vi "Write Cell font.vi"(8 "error in (no error)":errorcluster, 10 "Font":T1, 11 "DatagridElement in":refnum<class "DatagridElement.lvclass">) -> (0 "error out":errorcluster, 3 "DatagridElement out":refnum<class "DatagridElement.lvclass">)   [LabVIEW 2023, in "D Datagrid Library.lvlib" / "DatagridElement.lvclass"]
uses:
  DatagridElement.lvclass
  <vilib>/Utility/miscctls.llb/LVFontTypeDef.ctl
  DatagridElement.lvclass/DatagridElement.ctl
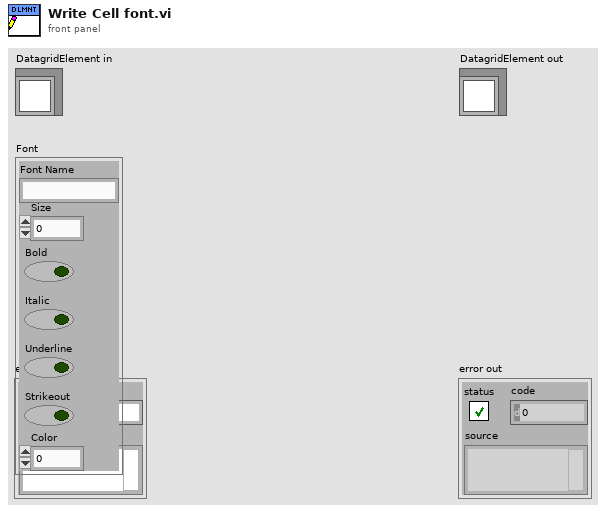
[diagram p1: front panel]
types:
  T1 = typedef "LVFontTypeDef.ctl" = cluster{"Font Name":string, "Size":u16, "Bold":bool, "Italic":bool, "Underline":bool, "Strikeout":bool, "Color":u32}
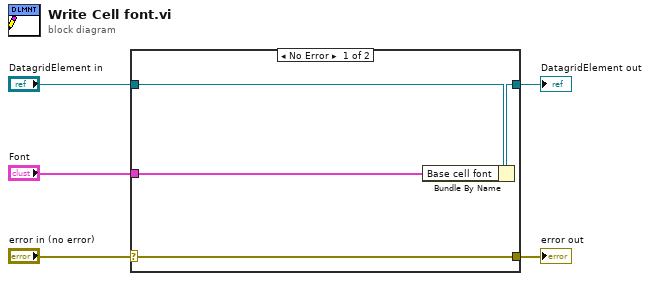
[diagram p0: block diagram]
diagram:
  n1 = case shown="No Error" "error in (no error)" {
    selector: "error in (no error)" -> [w9 w10]
    tunnel: [w9 w10] -> w4
    tunnel: [w7 w11] -> w2
    tunnel: "DatagridElement in" -> [w8 w11]
    tunnel: "Font" -> [w6 _]
    frame No Error {
      n2 = Bundle By Name(cluster=w8, "Base cell font"=w6) -> (w7:refnum<class "DatagridElement.lvclass">)
    }
    frame Error {
    }
  }
  "error out" <- w4
  "DatagridElement out" <- w2
